vi "Main - Seconds to Time (SubVI).vi"(11 "Seconds":dbl) -> (2 "Time string":string, 3 "Time":timestamp format="%<%H:%M:%S>T")   [LabVIEW 2019]
uses:
  <vilib>/Utility/miscctls.llb/LVDateTimeRec.ctl
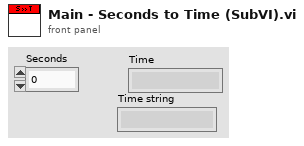
[diagram p1: front panel]
types:
  T1 = typedef "LVDateTimeRec.ctl" = cluster{"fractional second":dbl, "second":i32, "minute":i32, "hour":i32, "day of month":i32, "month":i32, "year":i32, "day of week":i32, "day of year":i32, "DST":i32}
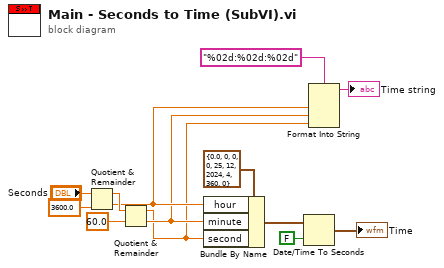
[diagram p0: block diagram]
diagram:
  n1 = Quotient & Remainder(x="Seconds", y=3600.0) -> (x-y*floor(x/y)=w9:dbl, floor(x/y)=w4:dbl)
  n2 = Quotient & Remainder(x=w9, y=60.0) -> (x-y*floor(x/y)=w2:dbl, floor(x/y)=w3:dbl)
  n3 = Bundle By Name(cluster=T1 {"fractional second"=0.0, "second"=0, "minute"=0, "hour"=0, "day of month"=25, "month"=12, "year"=2024, "day of week"=4, "day of year"=360, "DST"=0} ("date time rec"), "hour"=w4, "minute"=w3, "second"=w2) -> (w13:T1)
  n4 = Date/Time To Seconds(1:FALSE ("is UTC (F)"), 2:w13) -> (0:→"Time":timestamp)
  n5 = Format Into String(format string="%02d:%02d:%02d", w4, w3, w2) -> (resulting string=→"Time string":string)  [unwired: 2 in, 1 out]
